vi "Count Damaged Springs.vi"(11 "Record In":u8[](array[numeric])) -> (3 "Count Out":i64[](array[numeric]))   [LabVIEW 2021]
uses:
  <userlib>/_OpenG.lib/array/array.llb/Search 1D Array (U8)__ogtk.vi
  <userlib>/_OpenG.lib/array/array.llb/Search 1D Array (Boolean)__ogtk.vi
  <userlib>/_OpenG.lib/array/array.llb/Delete Elements from 1D Array (I32)__ogtk.vi
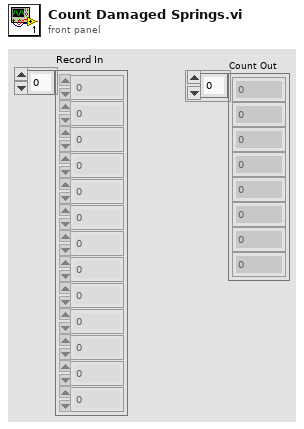
[diagram p1: front panel]
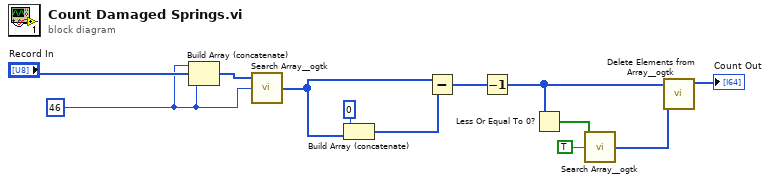
[diagram p0: block diagram]
diagram:
  w1 = u8 46 ("Element Data")
  n1 = Build Array (concatenate)(w1, "Record In", w1) -> (w3:u8[])
  n2 = call-poly <userlib>:"Search Array__ogtk.vi"("Array"=w3, "Element Data"=w1) -> ("Indices of Elements"=w9:i32[])  [unwired: 7 in]
  n3 = Build Array (concatenate)(0, w9) -> (w11:i32[])
  n4 = Subtract(x=w9, y=w11) -> (x-y=w10:i32[])
  n5 = Decrement(x=w10) -> (x-1=w6:i32[])
  n6 = Less Or Equal To 0?(x=w6) -> (x <= 0?=w8:bool[])
  n7 = call-poly <userlib>:"Search Array__ogtk.vi"("Array"=w8, "Element Data"=TRUE) -> ("Indices of Elements"=w5:i32[])  [unwired: 7 in]
  n8 = call-poly <userlib>:"Delete Elements from Array__ogtk.vi"("indices"=w5, "array"=w6) -> ("array w/ subset deleted"=→"Count Out":i32[])  [unwired: 8 in, 1 out]
